vi "Insert Item(s) (poly).vi"   [LabVIEW 2013, in "JSONtext.lvlib"]
uses:
  JSONtext.lvlib
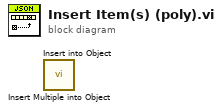
[diagram p0: block diagram]
diagram:
  n1 = call "Insert Multiple into Object.vi"() -> ()  [unwired: 8 in, 3 out]
  n2 = call "Insert into Object.vi"() -> ()  [unwired: 8 in, 3 out]
